vi "DB Tools Error Helper.vi"(8 "Overriding error or warning":errorcluster, 9 "source":string, 10 "code":i32, 11 "status":bool) -> (0 "error out":errorcluster)   [LabVIEW 2020, in "NI_Database_API.lvlib"]
doc: "Updates the error cluster to contain the specified error code and error source information."
uses:
  <vilib>/addons/database/NI_Database_API.lvlib
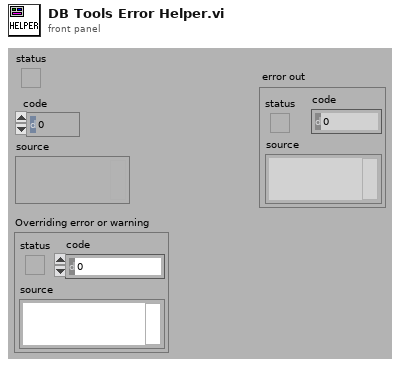
[diagram p1: front panel]
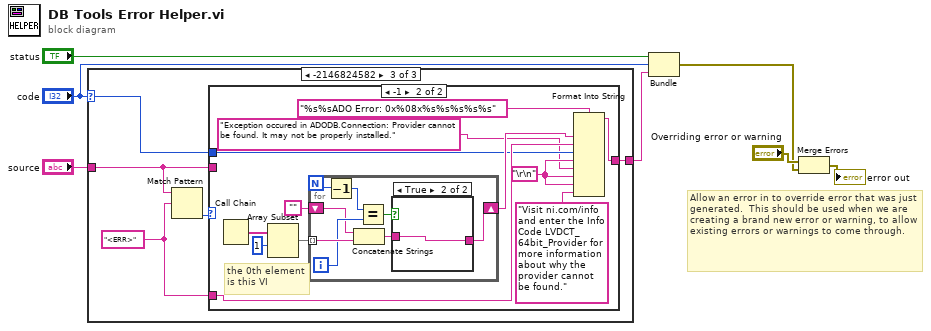
[diagram p0: block diagram]
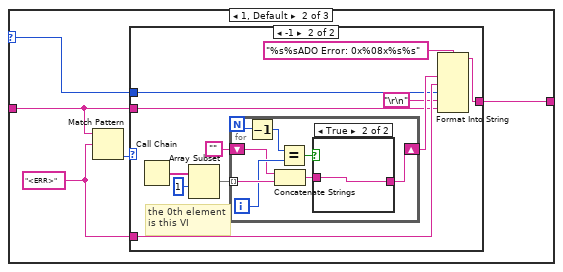
[diagram p3: hidden frame]
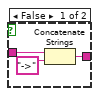
[diagram p5: hidden frame]
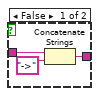
[diagram p7: hidden frame]
diagram:
  # "Allow an error in to override error that was just generated.  This should be used when we are creating a brand new error or warning, to allow existing errors or warnings to come through."
  n1 = case shown="-2146824582" "code" {
    selector: "code" -> [_ w9 w38]
    tunnel: [w8 w13 w42] -> w6
    tunnel: "source" -> [w8 w10 w39]
    frame 0 {
    }
    frame 1, Default {
      w12 = "<ERR>" ("Substring")
      n2 = Match Pattern(string=w10, regular expression=w12) -> (offset past match=w11:i32)  [unwired: 4 out]
      n3 = case shown="-1" w11 {
        tunnel: [w14 w19] -> w13
        tunnel: w10 -> [w14 w16]
        tunnel: w12 -> [_ w20]
        tunnel: w9 -> [_ w17]
        frame 0, Default {
        }
        frame -1 {
          # "the 0th element\nis this VI"
          n4 = Call Chain() -> (call chain=w22:string[])
          n5 = Array Subset(array=w22, index=1 ("Array Index")) -> (w24:string[])  [unwired: 1 in]
          n6 = for {
            N -> [w32]
            tunnel: w24 -> [w33] mode=indexing
            shift-right: [w26] -> w21
            shift-left: "" -> [w27]
            i -> [w30]
            n7 = Decrement(x=w32) -> (x-1=w31:i32)
            n8 = Concatenate Strings(w27, w33) -> (w28:string)
            n9 = Equal?(x=w31, y=w30) -> (x = y?=w29:bool)
            n10 = case shown="True" w29 {
              tunnel: w28 -> [w36 w37]
              tunnel: [w34 w37] -> w26
              frame False {
                n11 = Concatenate Strings(w36, "->" ("Substring")) -> (w34:string)
              }
              frame True {
              }
            }
          }
          n12 = Format Into String(format string="%s%sADO Error: 0x%08x%s%s", w21, w20, w17, "\r\n", w16) -> (resulting string=w19:string)  [unwired: 2 in, 1 out]
        }
      }
    }
    frame -2146824582 {
      w41 = "<ERR>" ("Substring")
      n13 = Match Pattern(string=w39, regular expression=w41) -> (offset past match=w40:i32)  [unwired: 4 out]
      n14 = case shown="-1" w40 {
        tunnel: [w43 w49] -> w42
        tunnel: w39 -> [w43 _]
        tunnel: w41 -> [_ w50]
        tunnel: w38 -> [_ w47]
        frame 0, Default {
        }
        frame -1 {
          w46 = "\r\n"
          # "the 0th element\nis this VI"
          n15 = Call Chain() -> (call chain=w52:string[])
          n16 = Array Subset(array=w52, index=1 ("Array Index")) -> (w54:string[])  [unwired: 1 in]
          n17 = for {
            N -> [w62]
            tunnel: w54 -> [w63] mode=indexing
            shift-right: [w56] -> w51
            shift-left: "" -> [w57]
            i -> [w60]
            n18 = Decrement(x=w62) -> (x-1=w61:i32)
            n19 = Concatenate Strings(w57, w63) -> (w58:string)
            n20 = Equal?(x=w61, y=w60) -> (x = y?=w59:bool)
            n21 = case shown="True" w59 {
              tunnel: w58 -> [w66 w67]
              tunnel: [w64 w67] -> w56
              frame False {
                n22 = Concatenate Strings(w66, "->" ("Substring")) -> (w64:string)
              }
              frame True {
              }
            }
          }
          n23 = Format Into String(format string="%s%sADO Error: 0x%08x%s%s%s%s%s", w51, w50, w47, w46, "Exception occured in ADODB.Connection: Provider cannot be found. It may not be properly installed." ("input 7"), w46, w46, "Visit ni.com/info and enter the Info Code LVDCT_64bit_Provider for more information about why the provider cannot be found." ("input 7")) -> (resulting string=w49:string)  [unwired: 2 in, 1 out]
        }
      }
    }
  }
  n24 = Bundle("status"="status", "code"="code", "source"=w6) -> (w1:errorcluster)  [unwired: 1 out]
  n25 = Merge Errors("Overriding error or warning", w1) -> (→"error out":errorcluster)
